vi "Configure Monitor Spectrum.vi"(0 "VISA resource name":refnum<visa-resource-name>, 1 "Averaging Method (0: Exponential)":i32(ring) items=["Exponential", "Repeat"], 5 "Average Count (0)":dbl, 7 "Frequency Span (26.5E+9 Hz)":dbl=26500000000.0 format="%^#_6g", 9 "Sweep Time (0.0146 s)":dbl=0.0146, 11 "error in (no error)":errorcluster) -> (4 "VISA resource name out":refnum<visa-resource-name>, 15 "error out":errorcluster)   [LabVIEW 2014, in "Agilent ESA PSA Series.lvlib"]
doc: "Configures the Monitor Spectrum measurement of the phase noise personality.\n\n<B>Note:</B> \n\nThis VI is only valid in Phase Noise personality. Use <B>Switch Personality</B> VI to switch to Phase Noise before calling this VI."
uses:
  Agilent ESA PSA Series.lvlib
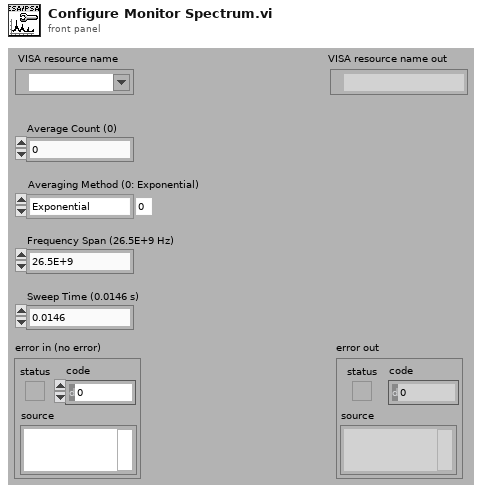
[diagram p1: front panel]
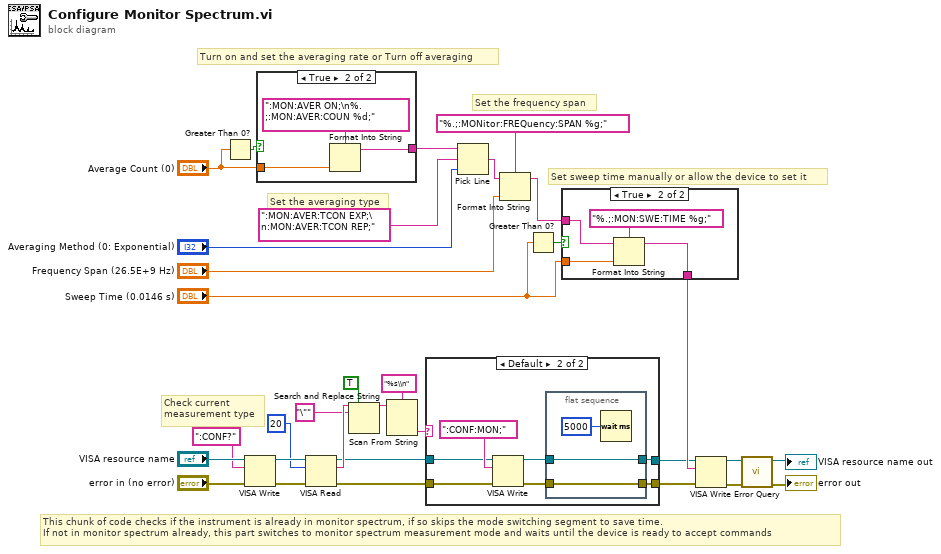
[diagram p0: block diagram]
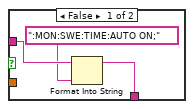
[diagram p3: hidden frame]
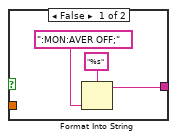
[diagram p4: hidden frame]
diagram:
  # "Check current\nmeasurement type"
  # "This chunk of code checks if the instrument is already in monitor spectrum, if so skips the mode switching segment to save time.\nIf not in monitor spectrum already, this part switches to monitor spectrum measurement mode and waits until the device is ready to accept commands"
  # "Set sweep time manually or allow the device to set it"
  # "Set the frequency span"
  # "Set the averaging type"
  # "Turn on and set the averaging rate or Turn off averaging"
  n1 = Greater Than 0?(x="Average Count (0)") -> (x > 0?=w28:bool)
  n2 = VISA Write(VISA resource name="VISA resource name", write buffer=":CONF?", error in (no error)="error in (no error)") -> (VISA resource name out=w8:refnum<visa-resource-name>, error out=w7:errorcluster)  [unwired: 1 out]
  n3 = case shown="True" w28 {
    tunnel: "Average Count (0)" -> [_ w38]
    tunnel: [w35 w36] -> w25
    frame False {
      n4 = Format Into String(format string="%s", ":MON:AVER OFF;" ("input 1")) -> (resulting string=w35:string)  [unwired: 2 in, 1 out]
    }
    frame True {
      n5 = Format Into String(format string=":MON:AVER ON;\n%.;:MON:AVER:COUN %d;", w38) -> (resulting string=w36:string)  [unwired: 2 in, 1 out]
    }
  }
  n6 = VISA Read(VISA resource name=w8, byte count=u32 20, error in (no error)=w7) -> (VISA resource name out=w1:refnum<visa-resource-name>, read buffer=w13:string, error out=w2:errorcluster)  [unwired: 1 out]
  n7 = Search and Replace String(replace all?=TRUE ("replace all? (F)"), input string=w13, search string="\"") -> (result string=w10:string)  [unwired: 5 in, 3 out]
  n8 = Scan From String(format string="%s\\n", input string=w10) -> (output 1=w5:string)  [unwired: 3 in, 3 out]
  n9 = case shown="Default" w5 {
    tunnel: [w39 w45] -> w3
    tunnel: [w40 w44] -> w4
    tunnel: w2 -> [w40 w41]
    tunnel: w1 -> [w39 w42]
    frame "MON", "MONitor" {
    }
    frame Default {
      n10 = VISA Write(VISA resource name=w42, write buffer=":CONF:MON;", error in (no error)=w41) -> (VISA resource name out=w47:refnum<visa-resource-name>, error out=w46:errorcluster)  [unwired: 1 out]
      n11 = flat-sequence {
        tunnel: w47 -> [w50]
        tunnel: w46 -> [w49]
        tunnel: [w50] -> w45
        tunnel: [w49] -> w44
        frame #0 {
          n12 = Wait (ms)(milliseconds to wait=u32 5000) -> ()  [unwired: 1 out]
        }
      }
    }
  }
  n13 = Pick Line(string ("")=w25, multi-line string=":MON:AVER:TCON EXP;\n:MON:AVER:TCON REP;", line index="Averaging Method (0: Exponential)") -> (output string=w23:string)
  n14 = Format Into String(format string="%.;:MONitor:FREQuency:SPAN %g;", initial string=w23, "Frequency Span (26.5E+9 Hz)") -> (resulting string=w19:string)  [unwired: 1 in, 1 out]
  n15 = Greater Than 0?(x="Sweep Time (0.0146 s)") -> (x > 0?=w20:bool)
  n16 = case shown="True" w20 {
    tunnel: w19 -> [w53 w56]
    tunnel: "Sweep Time (0.0146 s)" -> [_ w57]
    tunnel: [w51 w54] -> w17
    frame False {
      n17 = Format Into String(initial string=w53, ":MON:SWE:TIME:AUTO ON;" ("format string")) -> (resulting string=w51:string)  [unwired: 2 in, 1 out]
    }
    frame True {
      n18 = Format Into String(format string="%.;:MON:SWE:TIME %g;", initial string=w56, w57) -> (resulting string=w54:string)  [unwired: 1 in, 1 out]
    }
  }
  n19 = VISA Write(VISA resource name=w3, write buffer=w17, error in (no error)=w4) -> (VISA resource name out=w30:refnum<visa-resource-name>, error out=w29:errorcluster)  [unwired: 1 out]
  n20 = call "Error Query.vi"("error in (no error)"=w29, "VISA resource name"=w30) -> ("error out"=→"error out":errorcluster, "VISA resource name out"=→"VISA resource name out":refnum<visa-resource-name>)  [unwired: 6 in, 2 out]
